vi "FPGA Globals.vi"() -> ()   [LabVIEW 2015]
panel:
  out "bsLapReset":bool
  in  "stop":bool
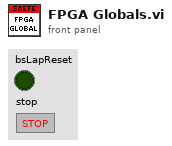
[diagram p1: front panel]
diagram:
